vi "fgv_parameter_sweep_array.vi"(7 "FGV Actions":T1, 8 "error in (no error)":errorcluster, 10 "Par. Sweep Array Size I/P":i32, 11 "Sweep Parameter Array":dbl[](array[numeric])) -> (0 "error out":errorcluster, 2 "Par. Sweep Array Size O/P":i32, 3 "Sweep Parameter Array":dbl[](array[numeric]))   [LabVIEW 2017]
uses:
  Typedefs/fgv_actions.ctl
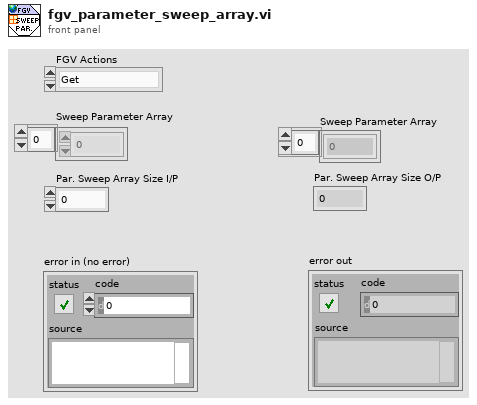
[diagram p1: front panel]
types:
  T1 = typedef "fgv_actions.ctl" = enum16{"Get", "Set"}
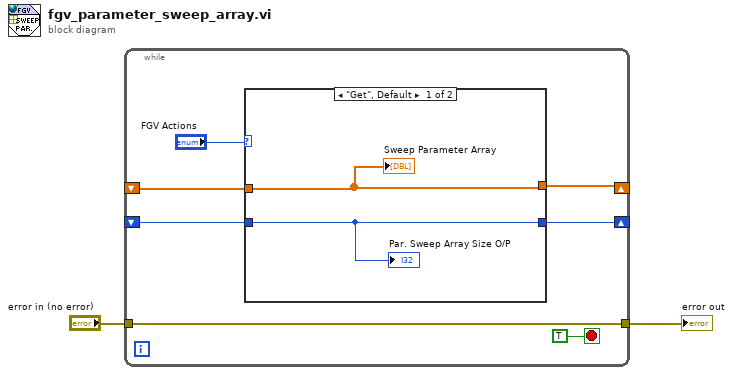
[diagram p0: block diagram]
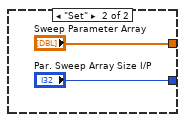
[diagram p2: hidden frame]
diagram:
  n1 = while {
    shift-right: [w7] -> _
    shift-left: _ -> [w6]
    tunnel: "error in (no error)" -> [w5]
    tunnel: [w5] -> w1
    shift-right: [w4] -> _
    shift-left: _ -> [w3]
    stop <- TRUE stop-if-true
    n2 = case shown="\"Get\", Default" "FGV Actions" {
      tunnel: [w11 "Sweep Parameter Array"] -> w7
      tunnel: w6 -> [w11 _]
      tunnel: [w10 "Par. Sweep Array Size I/P"] -> w4
      tunnel: w3 -> [w10 _]
      frame "Get", Default {
        "Sweep Parameter Array" <- w11
        "Par. Sweep Array Size O/P" <- w10
      }
      frame "Set" {
      }
    }
  }
  "error out" <- w1
